vi "Delete Tree Items.vi"(8 "error in (no error)":errorcluster, 9 "Items no longer in memory":string[](array[string]), 10 "Data Tree Ref":refnum<vi>, 11 "Data Value Reference in":refnum<data-value>) -> (0 "error out":errorcluster, 3 "TreeControl out":refnum<vi>)   [LabVIEW 2013, in "LVTM.lvlib"]
uses:
  LVTM.lvlib
  Controls_LVTM/SharedDataDVR.ctl
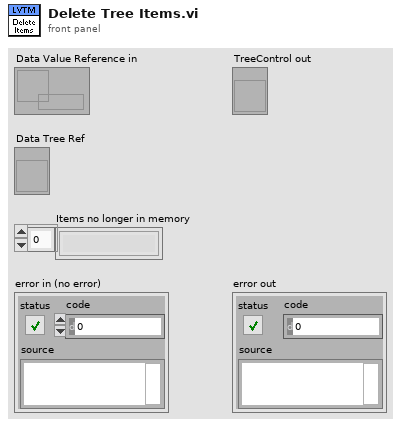
[diagram p1: front panel]
types:
  T1 = typedef "LVTM.lvlib/SharedDataDVR.ctl" = cluster{"App":refnum<vi>, "VIs":string[]}
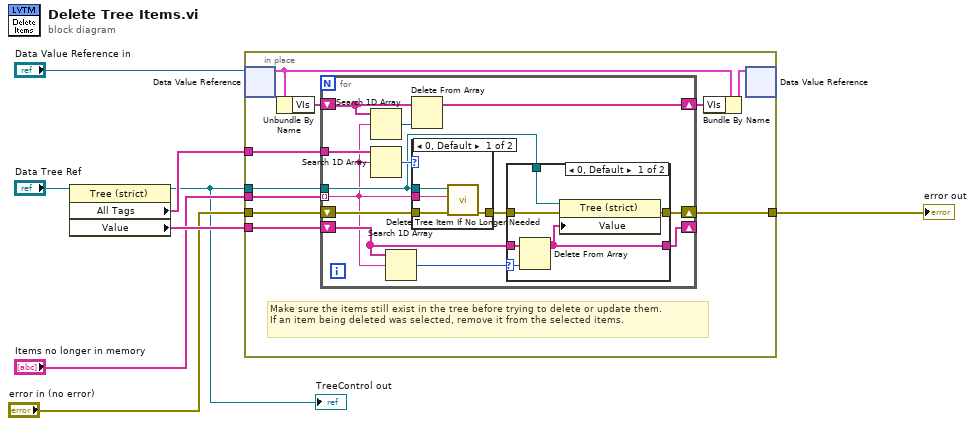
[diagram p0: block diagram]
diagram:
  n1 = property class="Tree (strict)"(reference="Data Tree Ref") -> (reference out=w1:refnum<vi>, "All Tags"=w8:string[], "Value"=w7:string[])  [unwired: 1 in, 1 out]
  "TreeControl out" <- w1
  n2 = in-place {
    in-place-border: w8 -> [w18]
    in-place-border: w1 -> [w17]
    in-place-border: [w16] -> w3
    in-place-border: "error in (no error)" -> [w15]
    in-place-border: "Items no longer in memory" -> [w14]
    in-place-border: w7 -> [w9]
    # "Make sure the items still exist in the tree before trying to delete or update them.\nIf an item being deleted was selected, remove it from the selected items."
    n3 = in-place-dvr #1("Data Value Reference in") -> (w13:T1)  [unwired: 1 out]
    n4 = Unbundle By Name(w13) -> ("VIs"=w11:string[])
    n5 = for {
      tunnel: w17 -> [w23]
      tunnel: w14 -> [w19] mode=indexing
      shift-right: [w24] -> w16
      shift-left: w15 -> [w31]
      tunnel: w18 -> [w30]
      shift-right: [w26] -> w10
      shift-left: w11 -> [w27]
      shift-right: [w22] -> _
      shift-left: w9 -> [w20]
      n6 = Search 1D Array(1D array=w27, element=w19) -> (index of element=w28:i32)  [unwired: 1 in]
      n7 = Search 1D Array(1D array=w30, element=w19) -> (index of element=w29:i32)  [unwired: 1 in]
      n8 = Search 1D Array(1D array=w20, element=w19) -> (index of element=w21:i32)  [unwired: 1 in]
      n9 = Delete From Array(array=w27, index=w28) -> (array with subset deleted=w26:string[])  [unwired: 1 in, 1 out]
      n10 = case shown="0, Default" w29 {
        tunnel: w23 -> [w43 _]
        tunnel: w31 -> [w42 w44]
        tunnel: [w41 w44] -> w25
        tunnel: w19 -> [w40 _]
        frame 0, Default {
          n11 = call "Delete Tree Item If No Longer Needed.vi"("error in"=w42, "Item Tag"=w40, "Tree Ref"=w43) -> ("error out"=w41:errorcluster)  [unwired: 8 in]
        }
        frame -1 {
        }
      }
      n12 = case shown="0, Default" w21 {
        selector: w21 -> [w32 _]
        tunnel: w20 -> [w37 w38]
        tunnel: w25 -> [w36 w39]
        tunnel: [w35 w39] -> w24
        tunnel: w23 -> [w34 _]
        tunnel: [w33 w38] -> w22
        frame 0, Default {
          n13 = Delete From Array(array=w37, index=w32) -> (array with subset deleted=w33:string[])  [unwired: 1 in, 1 out]
          n14 = property class="Tree (strict)"(reference=w34, error in=w36, "Value"=w33) -> (error out=w35:errorcluster)  [unwired: 1 out]
        }
        frame -1 {
        }
      }
    }
    n15 = Bundle By Name(cluster=w13, "VIs"=w10) -> (w12:T1)
    n16 = in-place-dvr #1(w12) -> ()  [unwired: 2 out]
  }
  "error out" <- w3
